vi "D-O Module (Main).vi"(7 "Name of Parent Panel":string="Main.vi", 9 "New Center Coords":T1={"Horizontal"=470, "Vertical"=200}, 10 "Config":variant, 11 "Main UI Message Queue":refnum<queue>) -> ()   [LabVIEW 2018, in "D-O Module.lvlib"]
doc: "This Continuous Measurement sample project is based on the Queued Message Handler template.\n\nThe Event Handling Loop generates messages based on user interface actions.\n\nThe Message Handling Loop processes messages generated by the Event Handling Loop, or by other messages. There are also Acquisition and Logging message handling loop subVIs, and a chart updating loop."
uses:
  D-O Module.lvlib
  support/Message Queue/Message Cluster.ctl
  <vilib>/Utility/miscctls.llb/LVPoint32TypeDef.ctl
  controls/UI Data.ctl
  controls/UI State.ctl
  D-O Module State Cluster.ctl
  D-O Module Config Cluster.ctl
  Valve Clusters.ctl
  D-O Module Settings Cluster.ctl
  D-O Device Settings Cluster.ctl
  VICI Electronic Actuator/VICI Electronic Actuator Settings.ctl
  Measure Instrument/State Enum.ctl
  D-O Module Display.ctl
  Sequencing/Squence Update Cluster.ctl
  support/Message Queue/Enqueue Message (Single).vi
  <vilib>/Utility/error.llb/Error Cluster From Error Code.vi
  <vilib>/ErrorRing/Error Ring.xnode
  support/User Event - Stop/User Event - Stop.lvlib
  support/Support Library.lvlib
  support/Message Queue/Message Queue.lvlib
  Measure Instrument/D-O Module Engine.lvlib
  Measure Instrument/Feed Module Engine.lvlib
  Sequencing/Sequencing Library.lvlib
  D-O Settings Dialog.vi
  support/Command Log VIs/Command Logging.lvlib
  DIO Valve/VICI Electronic Actuator.lvlib
panel:
  out "Sequence Started":bool
  in  "Settings Button":bool
  out "ScanCode":i16
  out "Ring":u16(ring)=2
  out "Log File path":path
  out "Status":string
  in  "Exit":bool
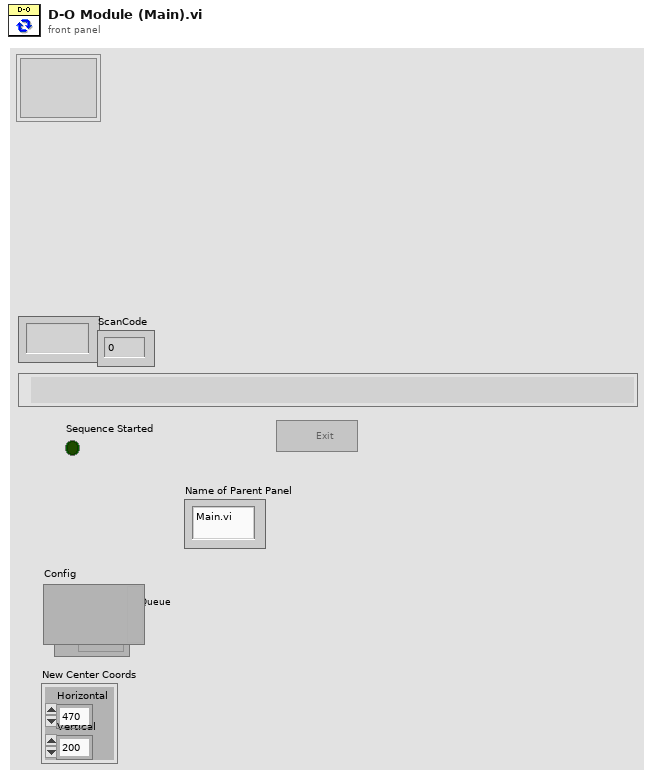
[diagram p1: front panel]
types:
  T1 = typedef "LVPoint32TypeDef.ctl" = cluster{"Horizontal":i32, "Vertical":i32}
  T2 = typedef "D-O Module.lvlib/D-O Module Config Cluster.ctl" = cluster{"GUID":string, "Drop Coords":T1, "Process Name":string, "Queue Name":string, "Settings":T3, "Load Count":i32}
  T3 = typedef "D-O Module.lvlib/Valve Clusters.ctl" = cluster{"Valve Settings":T4, "Valve Type":enum16{"Default", "Digital Output Valve", "VICI Electronic Actuator"}, "Time On (Sec)":dbl, "Time Off (Sec)":dbl, "Run?":bool}
  T4 = typedef "D-O Module.lvlib/D-O Module Settings Cluster.ctl" = cluster{"D-O Settings":T5, "VICI Electronic Actuator":T6}
  T5 = typedef "D-O Module.lvlib/D-O Device Settings Cluster.ctl" = cluster{"DAQmx Task Name":refnum<k21>, "Output Channel":u16, "Output Channel Names":string[]}
  T6 = typedef "VICI Electronic Actuator.lvlib/VICI Electronic Actuator Settings.ctl" = cluster{"VISA resource name":refnum<visa-resource-name>, "Mode":enum16{"Two Positions With Stops", "Two Positions Without Stops", "Mutiposition"}, "Simulated":bool}
  T7 = typedef "D-O Module.lvlib/D-O Module State Cluster.ctl" = cluster{"D-O Module Config":T2, "State":T8, "Start Time":timestamp, "Current Time":timestamp, "First Iteration":bool, "Data":cluster{"Valve State":T4}, "Process Name":string, "Queue Name":string, "Program On?":bool}
  T8 = typedef "Feed Module.lvlib/Feed Module Engine.lvlib/State Enum.ctl" = enum16{"Measuring", "Idle", "Paused"}
  T9 = typedef "UI State.ctl" = enum16{"Idle", "Acquiring and Logging", "Waiting for Exit", "Waiting for Exit (Acq Stopped)", "Waiting for Exit (Log Stopped)", "Waiting for Stop", "Waiting for Stop (Acq Stopped)", "Waiting for Stop (Log Stopped)"}
  T10 = typedef "UI Data.ctl" = cluster{"Start Ref":refnum<vi>, "Trigger Ref":refnum<vi>, "Stop Ref":refnum<vi>, "Settings Ref":refnum<vi>, "Status Ref":refnum<vi>, "Exit Ref":refnum<vi>, "Data Ref":refnum<vi>}
  T11 = typedef "D-O Module.lvlib/All Message Queues.ctl" = cluster{"Engine":refnum<queue>, "D-O UI":refnum<queue>, "D-O Engine":refnum<queue>, "D-O Display":refnum<queue>}
  T12 = typedef "Sequencing Library.lvlib/Squence Update Cluster.ctl" = cluster{"Auto?":bool, "Manual Entry":dbl, "Setpoint":dbl}
  T13 = enum8{"Enabled", "Disabled", "Disabled and Grayed Out"}
  T14 = typedef "D-O Module.lvlib/D-O Module Display.ctl" = cluster{"D-O State ":u16, "Cycle Period":dbl}
  T15 = cluster{"Shift":bool, "Ctrl":bool, "Alt":bool, "Cmd":bool, "Opt":bool}
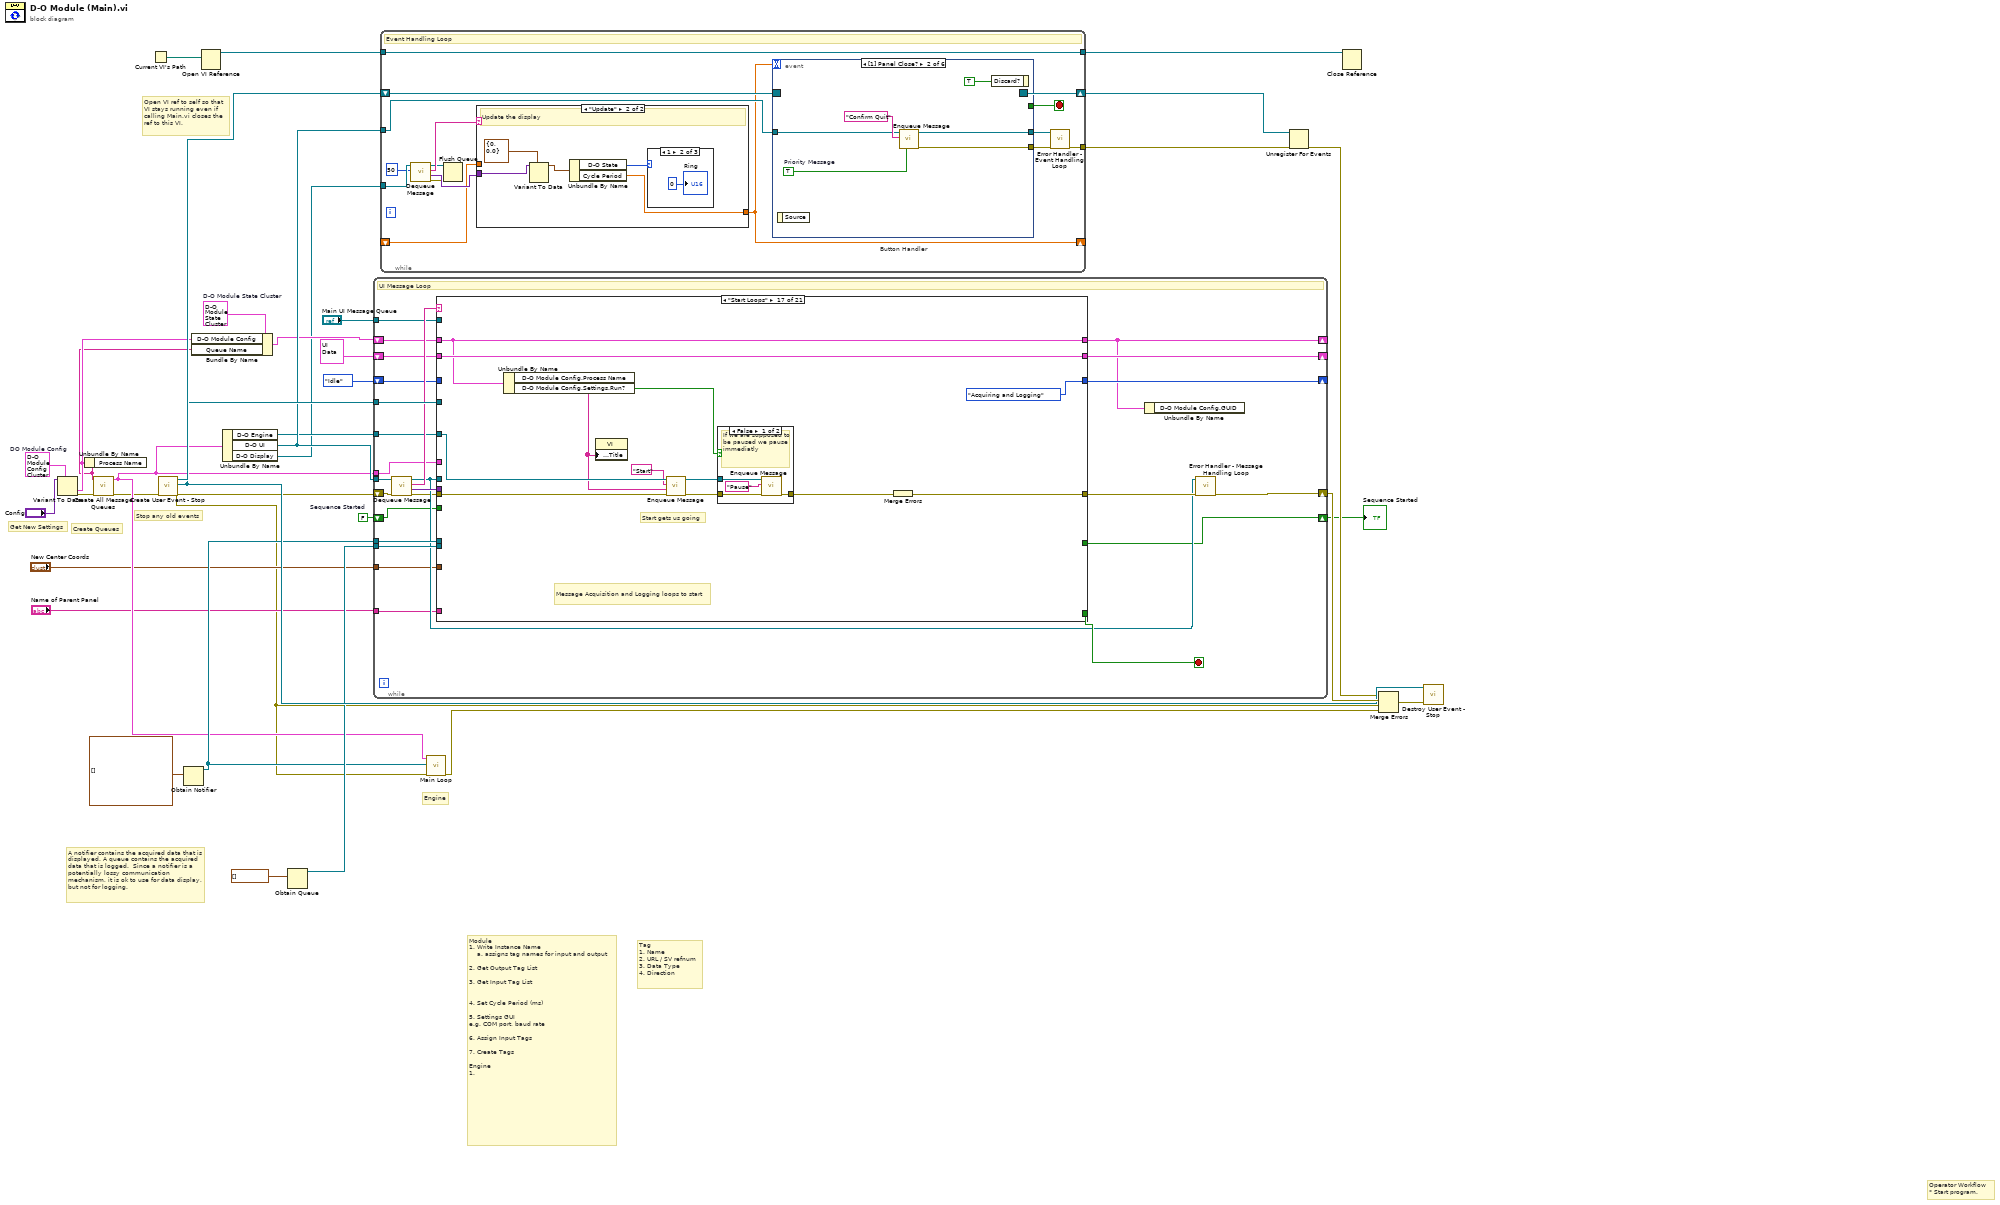
[diagram p0: block diagram]
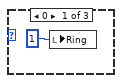
[diagram p3: hidden frame]
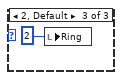
[diagram p4: hidden frame]
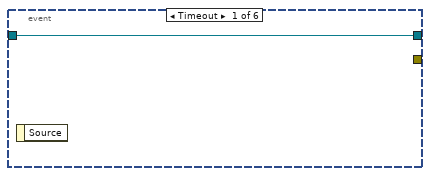
[diagram p5: hidden frame]
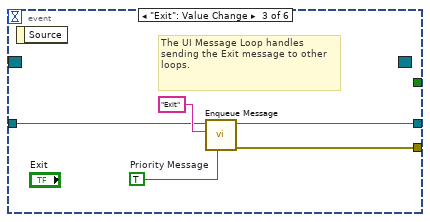
[diagram p6: hidden frame]
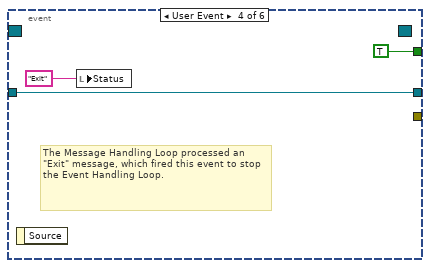
[diagram p7: hidden frame]
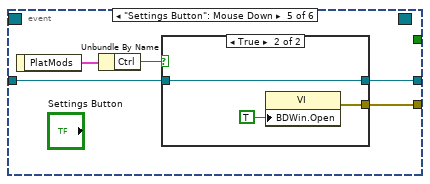
[diagram p8: hidden frame]
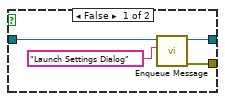
[diagram p9: hidden frame]
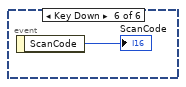
[diagram p10: hidden frame]
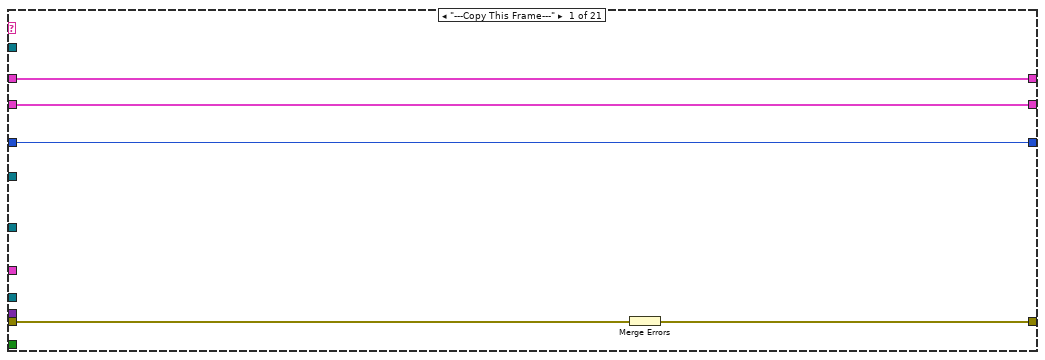
[diagram p11: hidden frame]
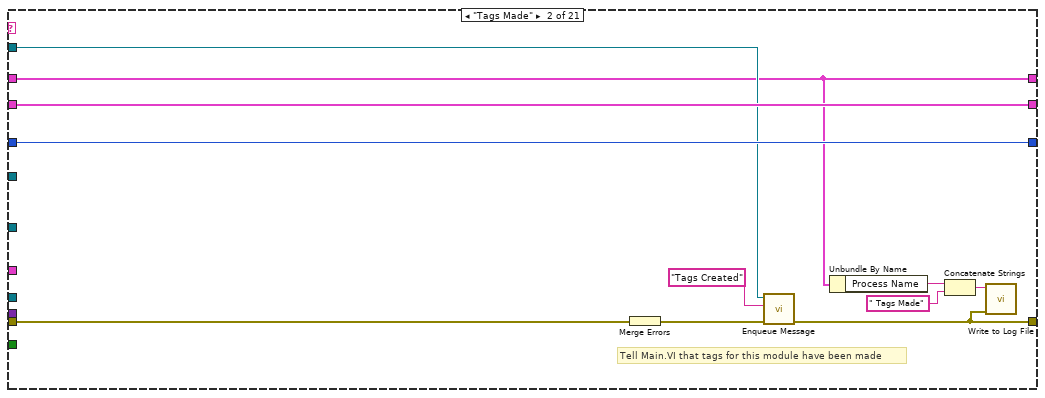
[diagram p12: hidden frame]
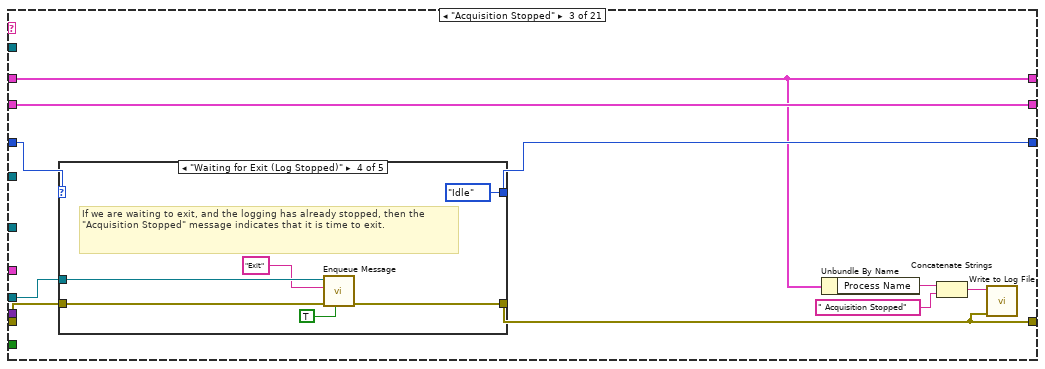
[diagram p13: hidden frame]
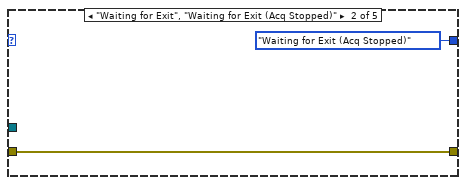
[diagram p15: hidden frame]
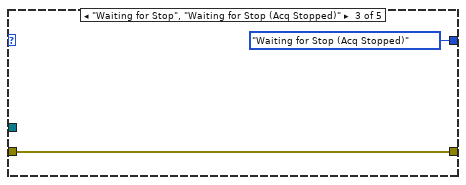
[diagram p16: hidden frame]
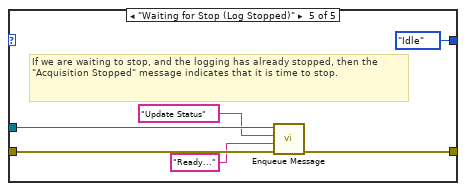
[diagram p17: hidden frame]
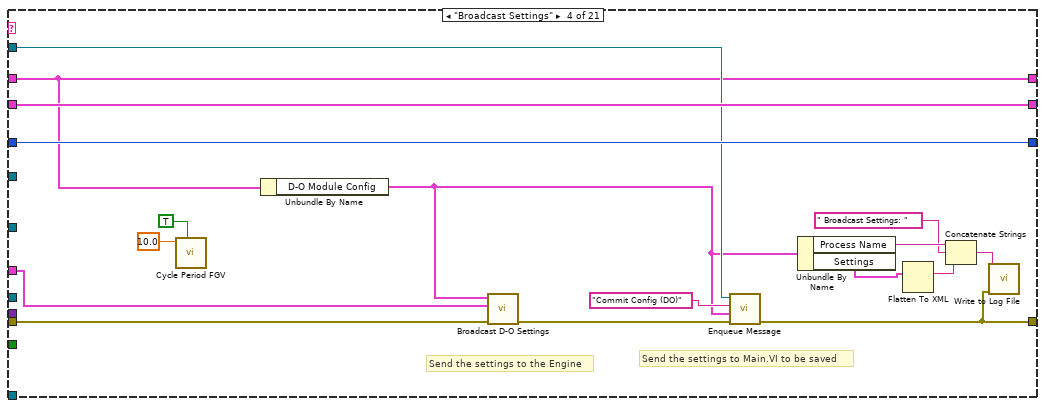
[diagram p18: hidden frame]
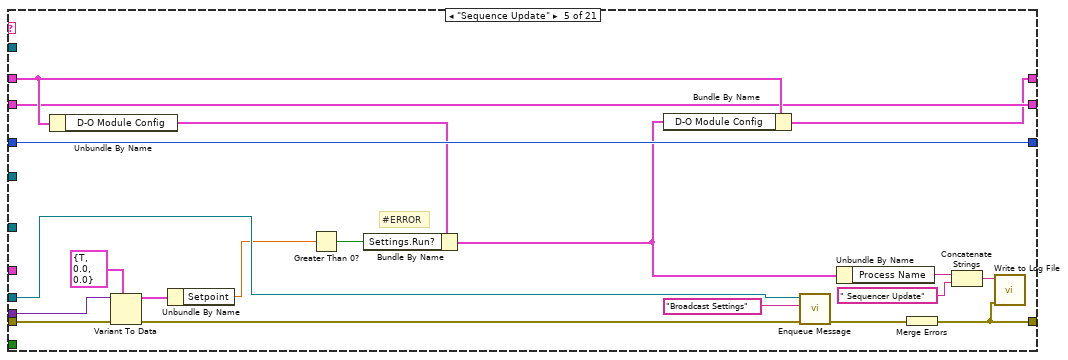
[diagram p19: hidden frame]
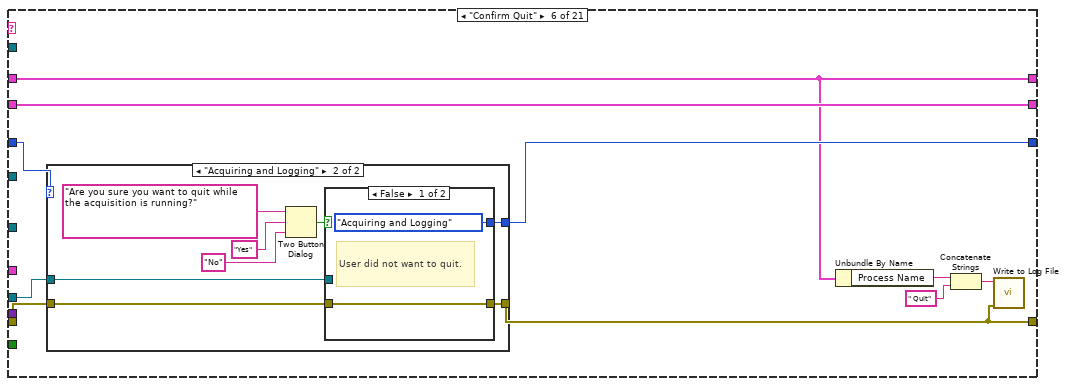
[diagram p20: hidden frame]
diagram:
  w7 = FALSE  # Sequence Started
  w6 = T2 {"GUID"="", "Drop Coords"={"Horizontal"=0, "Vertical"=0}, "Process Name"="", "Queue Name"="", "Settings"={"Valve Settings"={"D-O Settings"={"DAQmx Task Name"="", "Output Channel"=0, "Output Channel Names"=[]}, "VICI Electronic Actuator"={"VISA resource name"="", "Mode"=enum."Two Positions With Stops", "Simulated"=FALSE}}, "Valve Type"=enum."Default", "Time On (Sec)"=0.0, "Time Off (Sec)"=0.0, "Run?"=FALSE}, "Load Count"=0}  # DO Module Config
  w14 = T7 {"D-O Module Config"={"GUID"="", "Drop Coords"={"Horizontal"=0, "Vertical"=0}, "Process Name"="", "Queue Name"="", "Settings"={"Valve Settings"={"D-O Settings"={"DAQmx Task Name"="", "Output Channel"=0, "Output Channel Names"=[]}, "VICI Electronic Actuator"={"VISA resource name"="", "Mode"=enum."Two Positions With Stops", "Simulated"=FALSE}}, "Valve Type"=enum."Digital Output Valve", "Time On (Sec)"=0.0, "Time Off (Sec)"=0.0, "Run?"=FALSE}, "Load Count"=0}, "State"=enum."Idle", "Start Time"=timestamp(0 s since 1904-01-01), "Current Time"=timestamp(0 s since 1904-01-01), "First Iteration"=FALSE, "Data"={"Valve State"={"D-O Settings"={"DAQmx Task Name"="", "Output Channel"=0, "Output Channel Names"=[]}, "VICI Electronic Actuator"={"VISA resource name"="", "Mode"=enum."Two Positions With Stops", "Simulated"=FALSE}}}, "Process Name"="", "Queue Name"="", "Program On?"=FALSE}  # D-O Module State Cluster
  # "Stop any old events"
  # "Create Queues"
  # "Get New Settings"
  # "Open VI ref to self so that\nVI stays running even if\ncalling Main.vi closes the\nref to this VI."
  # "Engine"
  # "Operator Workflow\n* Start program."
  # "Module \n1. Write Instance Name\n    a. assigns tag names for input and output\n\n2. Get Output Tag List\n\n3. Get Input Tag List\n\n\n4. Set Cycle Period (ms)\n\n5. Settings GUI\ne.g. COM port, baud rate\n\n6. Assign Input Tags\n\n7. Create Tags\n\nEngine\n1."
  # "Tag\n1. Name\n2. URL / SV refnum\n3. Data Type\n4. Direction"
  # "A notifier contains the acquired data that is displayed. A queue contains the acquired data that is logged.  Since a notifier is a potentially lossy communication mechanism, it is ok to use for data display, but not for logging."
  n1 = Variant To Data(type=w6, Variant="Config") -> (data=w5:T2, error out=w4:errorcluster)  [unwired: 1 in]
  n2 = Unbundle By Name(w5) -> ("Process Name"=w1:string)
  n3 = call "Create All Message Queues.vi"("error in (no error)"=w4, "Process Name"=w1) -> ("error out"=w3:errorcluster, "Message Queues"=w11:T11)  [unwired: 8 in]
  n4 = Current VI's Path() -> (path=w17:path)
  n5 = call "Create User Event - Stop.vi"("error in (no error)"=w3) -> ("error out"=w2:errorcluster, "User Event - Stop"=w31:refnum<user-event>, "Stop Event Registration Refnum"=w32:refnum<event-registration>)  [unwired: 8 in]
  n6 = Obtain Notifier(notification data type=waveform(dbl)[] []) -> (notifier out=w20:refnum<notifier>)  [unwired: 3 in, 2 out]
  n7 = Bundle By Name(cluster=w14, "D-O Module Config"=w5, "Queue Name"=w1) -> (w16:T7)
  n8 = Open VI Reference(vi path=w17) -> (vi reference=w18:refnum<vi>)  [unwired: 5 in, 1 out]
  n9 = Unbundle By Name(w11) -> ("D-O Engine"=w23:refnum<queue>, "D-O UI"=w27:refnum<queue>, "D-O Display"=w13:refnum<queue>)
  n10 = Obtain Queue(element data type=waveform(dbl)[] []) -> (queue out=w22:refnum<queue>)  [unwired: 4 in, 2 out]
  n11 = while {
    tunnel: w27 -> [w55]
    tunnel: w31 -> [w59]
    shift-right: [w49] -> w35
    shift-left: w2 -> [w58]
    shift-right: [w36] -> _
    shift-left: w16 -> [w43]
    shift-right: [w53] -> _
    shift-left: T10 {"Start Ref"=refnum, "Trigger Ref"=refnum, "Stop Ref"=refnum, "Settings Ref"=refnum, "Status Ref"=refnum, "Exit Ref"=refnum, "Data Ref"=refnum} ("Measurement UI Controls") -> [w54]
    tunnel: w20 -> [w52]
    tunnel: w22 -> [w51]
    shift-right: [w46] -> _
    shift-left: UI_State."Idle" ("UI State") -> [w47]
    tunnel: w23 -> [w45]
    tunnel: "Main UI Message Queue" -> [w42]
    tunnel: w11 -> [w41]
    tunnel: "New Center Coords" -> [w40]
    tunnel: "Name of Parent Panel" -> [w39]
    shift-right: [w38] -> w8
    shift-left: w7 -> [w37]
    stop <- w60 stop-if-true
    # "UI Message Loop"
    n12 = call "Dequeue Message.vi"("error in (no error)"=w58, "Message Queue"=w55) -> ("error out"=w44:errorcluster, "Message Data"=w56:variant, "Message"=w57:string, "dup Message Queue"=w48:refnum<queue>)  [unwired: 6 in]
    n13 = case "Message Cases" shown="\"Start Loops\"" w57 {
      selector: w57 -> [_ _ _ _ _ _ _ _ _ _ _ _ _ _ _ _ _ _ _ _ w480]
      tunnel: w48 -> [_ _ w82 _ w137 w149 _ w207 w222 w249 _ w283 w302 w308 w344 w376 _ _ w436 _ _]
      tunnel: w44 -> [w65 w76 w83 w118 w135 w148 w175 w188 w226 w253 w268 w278 w299 w310 w342 w375 w402 w418 w438 w471 _]
      tunnel: [w64 w70 w81 w111 w123 w143 w176 w182 w216 w228 w268 w273 w294 w309 w333 w364 w406 w416 w433 w472 w483] -> w50
      tunnel: [_ _ _ _ _ _ _ _ _ TRUE _ _ _ _ _ _ _ _ _ _ _] -> w60
      tunnel: w56 -> [_ _ _ _ w138 _ w178 _ w225 w237 _ _ _ _ _ _ _ _ _ w470 _]
      tunnel: w59 -> [_ _ _ _ _ _ _ _ _ w252 _ _ _ _ _ _ _ _ _ _ _]
      tunnel: w43 -> [w61 w66 w77 w115 w140 w142 w173 w186 w213 w229 w259 w269 w301 w307 w338 w371 w400 w412 w440 w461 w478]
      tunnel: w54 -> [w63 w75 w86 w121 w139 w151 w180 w204 w227 w250 w267 w279 w306 w313 w339 w372 w405 w423 w456 w467 w485]
      tunnel: [w63 w75 w86 w121 w139 w151 w180 w204 w227 w250 w266 w279 w306 w313 w339 w372 w405 w423 w456 w467 w485] -> w53
      tunnel: w52 -> [_ _ _ _ _ _ _ _ _ w248 _ _ _ _ _ _ _ _ _ _ _]
      tunnel: w51 -> [_ _ _ _ _ _ _ _ _ w244 _ _ _ _ _ _ _ _ _ _ _]
      tunnel: w47 -> [w62 w74 w85 w120 w141 w150 w174 w193 w217 _ _ _ w305 w312 _ _ _ _ w445 w462 w484]
      tunnel: [w62 w74 w84 w120 w141 w147 w174 w194 w217 UI_State."Idle" ("UI State") UI_State."Idle" ("UI State") UI_State."Idle" ("UI State") w305 w311 UI_State."Acquiring and Logging" ("UI State") UI_State."Acquiring and Logging" ("UI State") UI_State."Acquiring and Logging" ("UI State") UI_State."Acquiring and Logging" ("UI State") w446 w462 w484] -> w46
      tunnel: w45 -> [_ _ _ _ _ _ _ w192 _ w236 _ _ _ _ _ _ w403 w421 w444 _ _]
      tunnel: w42 -> [_ w71 _ w117 _ _ _ _ _ w238 _ _ _ _ _ _ _ _ _ _ _]
      tunnel: [w61 w66 w77 w115 w136 w142 w173 w181 w213 w229 w259 w269 w290 w307 w332 w361 w400 w412 w429 w461 w478] -> w36
      tunnel: w41 -> [_ _ _ w113 _ _ _ _ _ _ _ _ w296 _ _ _ _ _ _ _ _]
      tunnel: w40 -> [_ _ _ _ _ _ _ _ _ _ _ w276 _ _ _ _ _ _ _ _ _]
      tunnel: w39 -> [_ _ _ _ _ _ _ _ _ _ _ w275 _ _ _ _ _ _ _ _ _]
      tunnel: [_ _ _ _ _ _ _ _ _ _ _ _ _ _ _ w369 _ _ _ _ _] -> w38
      tunnel: w37 -> [_ _ _ _ _ _ _ _ _ _ _ _ _ _ _ w365 _ _ _ _ _]
      frame "---Copy This Frame---" {
        # "Duplicate this frame when creating new messages.  Change this comment in the duplicated frame to describe this message."
        n14 = Merge Errors(w65) -> (w64:errorcluster)
      }
      frame "Tags Made" {
        # "Tell Main.VI that tags for this module have been made"
        # "Duplicate this frame when creating new messages.  Change this comment in the duplicated frame to describe this message."
        n15 = Merge Errors(w76) -> (w72:errorcluster)
        n16 = call-poly "Enqueue Message.vi"("error in (no error)"=w72, "Message"="Tags Created", "Message Queue"=w71) -> ("error out"=w70:errorcluster)  [unwired: 7 in, 1 out]
        n17 = Unbundle By Name(w66) -> ("Process Name"=w69:string)
        n18 = Concatenate Strings(w69, " Tags Made" ("text")) -> (w67:string)
        n19 = call "Write to Log File.vi"("error in"=w70, "text"=w67) -> ()  [unwired: 9 in, 1 out]
      }
      frame "Acquisition Stopped" {
        # "Logic for determining what action to take when the acquisition has stopped."
        n20 = case shown="\"Waiting for Exit (Log Stopped)\"" w85 {
          selector: w85 -> [w88 _ _ _ _]
          tunnel: [w88 UI_State."Waiting for Exit (Acq Stopped)" ("UI State") UI_State."Waiting for Stop (Acq Stopped)" ("UI State") UI_State."Idle" ("UI State") UI_State."Idle" ("UI State")] -> w84
          tunnel: w83 -> [w87 w89 w91 w97 w103]
          tunnel: [w87 w89 w91 w96 w102] -> w81
          tunnel: w82 -> [_ _ _ w95 w101]
          frame Default {
          }
          frame "Waiting for Exit", "Waiting for Exit (Acq Stopped)" {
          }
          frame "Waiting for Stop", "Waiting for Stop (Acq Stopped)" {
          }
          frame "Waiting for Exit (Log Stopped)" {
            # "If we are waiting to exit, and the logging has already stopped, then the \"Acquisition Stopped\" message indicates that it is time to exit."
            n21 = call-poly "Enqueue Message.vi"("Priority Message? (F)"=TRUE, "error in (no error)"=w97, "Message"="Exit", "Message Queue"=w95) -> ("error out"=w96:errorcluster)  [unwired: 6 in, 1 out]
          }
          frame "Waiting for Stop (Log Stopped)" {
            # "If we are waiting to stop, and the logging has already stopped, then the \"Acquisition Stopped\" message indicates that it is time to stop."
            n22 = call-poly "Enqueue Message.vi"("error in (no error)"=w103, "Message Data"="Ready..." ("Message"), "Message"="Update Status", "Message Queue"=w101) -> ("error out"=w102:errorcluster)  [unwired: 6 in, 1 out]
          }
        }
        n23 = Unbundle By Name(w77) -> ("Process Name"=w80:string)
        n24 = Concatenate Strings(w80, " Acquisition Stopped" ("text")) -> (w78:string)
        n25 = call "Write to Log File.vi"("error in"=w81, "text"=w78) -> ()  [unwired: 9 in, 1 out]
      }
      frame "Broadcast Settings" {
        # "Send the settings to Main.VI to be saved"
        # "Send the settings to the Engine"
        # "Send the 'Update Settings' message to the Logging and Acquisition message loops."
        n26 = call "Cycle Period FGV.vi"("Write"=TRUE, "Cycle Period In (ms)"=10.0) -> ()  [unwired: 8 in, 2 out]
        n27 = Unbundle By Name(w115) -> ("D-O Module Config"=w107:T2)
        n28 = call "Broadcast D-O Settings.vi"("error in (no error)"=w118, "Message Queues"=w113, "D-O Module Config"=w107) -> ("error out"=w116:errorcluster)  [unwired: 8 in]
        n29 = call-poly "Enqueue Message.vi"("error in (no error)"=w116, "Message Data"=w107, "Message"="Commit Config (DO)", "Message Queue"=w117) -> ("error out"=w111:errorcluster)  [unwired: 6 in, 1 out]
        n30 = Unbundle By Name(w107) -> ("Process Name"=w110:string, "Settings"=w105:T3)
        n31 = Flatten To XML(anything=w105) -> (xml string=w106:string)
        n32 = Concatenate Strings(w110, " Broadcast Settings: " ("text"), w106) -> (w108:string)
        n33 = call "Write to Log File.vi"("error in"=w111, "text"=w108) -> ()  [unwired: 9 in, 1 out]
      }
      frame "Sequence Update" {
        # "#ERROR"
        n34 = Unbundle By Name(w140) -> ("D-O Module Config"=w134:T2)
        n35 = Variant To Data(error in=w135, type=T12 {"Auto?"=TRUE, "Manual Entry"=0.0, "Setpoint"=0.0} ("Cluster"), Variant=w138) -> (data=w132:T12, error out=w129:errorcluster)
        n36 = Unbundle By Name(w132) -> ("Setpoint"=w127:dbl)
        n37 = Greater Than 0?(x=w127) -> (x > 0?=w128:bool)
        n38 = Bundle By Name(cluster=w134, "Settings.Run?"=w128) -> (w122:T2)
        n39 = Bundle By Name(cluster=w140, "D-O Module Config"=w122) -> (w136:T7)
        n40 = call-poly "Enqueue Message.vi"("error in (no error)"=w129, "Message"="Broadcast Settings", "Message Queue"=w137) -> ("error out"=w131:errorcluster)  [unwired: 7 in, 1 out]
        n41 = Unbundle By Name(w122) -> ("Process Name"=w126:string)
        n42 = Merge Errors(w131) -> (w123:errorcluster)
        n43 = Concatenate Strings(w126, " Sequencer Update" ("text")) -> (w124:string)
        n44 = call "Write to Log File.vi"("error in"=w123, "text"=w124) -> ()  [unwired: 9 in, 1 out]
      }
      frame "Confirm Quit" {
        # "Confirm Quit - Message that can confirm whether or not the user wants to exit the application."
        n45 = case shown="\"Acquiring and Logging\"" w150 {
          tunnel: w149 -> [w156 w162]
          tunnel: w148 -> [w155 w160]
          tunnel: [w152 w159] -> w143
          tunnel: [UI_State."Idle" ("UI State") w158] -> w147
          frame Default {
            # "If 'Confirm Quit' comes in while the system is idle, there is no need for a confirmation message."
            n46 = call-poly "Enqueue Message.vi"("Priority Message? (F)"=TRUE, "error in (no error)"=w155, "Message"="Exit", "Message Queue"=w156) -> ("error out"=w152:errorcluster)  [unwired: 6 in, 1 out]
          }
          frame "Acquiring and Logging" {
            n47 = Two Button Dialog(message="Are you sure you want to quit while the acquisition is running?" ("Confirm Quit Message"), 1:"No" ("No"), 2:"Yes" ("Yes")) -> (T button?=w161:bool)
            n48 = case shown="False" w161 {
              tunnel: w162 -> [_ w172]
              tunnel: w160 -> [w166 w171]
              tunnel: [w166 w170] -> w159
              tunnel: [UI_State."Acquiring and Logging" ("UI State") UI_State."Waiting for Exit" ("UI State")] -> w158
              frame False {
                # "User did not want to quit."
              }
              frame True {
                n49 = call-poly "Enqueue Message.vi"("error in (no error)"=w171, "Message"="Stop", "Message Queue"=w172) -> ("error out"=w170:errorcluster)  [unwired: 7 in, 1 out]
              }
            }
          }
        }
        n50 = Unbundle By Name(w142) -> ("Process Name"=w146:string)
        n51 = Concatenate Strings(w146, " Quit" ("text")) -> (w144:string)
        n52 = call "Write to Log File.vi"("error in"=w143, "text"=w144) -> ()  [unwired: 9 in, 1 out]
      }
      frame "Display Log File Path" {
        n53 = Variant To Data(error in=w175, type=path "", Variant=w178) -> (data=→"Log File path":path, error out=w176:errorcluster)
      }
      frame "E-Stop" {
        # "Pause the DO when E-Stop is sent"
        # "Message Acquisition and Logging loops to stop"
        # "Enable: Start, Exit, Settings\nDisable: Stop"
        # "Stop the pumps."
        n54 = Unbundle By Name(w204) -> ("Trigger Ref"=w195:refnum<vi>, "Stop Ref"=w196:refnum<vi>, "Start Ref"=w199:refnum<vi>, "Exit Ref"=w198:refnum<vi>, "Settings Ref"=w197:refnum<vi>)
        n55 = call-poly "Enqueue Message.vi"("error in (no error)"=w188, "Message Data"="Ready..." ("Ready..."), "Message"="Update Status", "Message Queue"=w207) -> ("error out"=w190:errorcluster)  [unwired: 6 in, 1 out]
        n56 = Build Array(w199, w198, w197) -> (w202:refnum<vi>[])
        n57 = Build Array(w195, w196) -> (w201:refnum<vi>[])
        n58 = call-poly "Enqueue Message.vi"("error in (no error)"=w190, "Message"="Pause", "Message Queue"=w192) -> ("error out"=w189:errorcluster)  [unwired: 7 in, 1 out]
        n59 = call "Set Enable State on Multiple Controls.vi"("Enable?"=FALSE, "Controls"=w201) -> ()  [unwired: 10 in]
        n60 = call "Set Enable State on Multiple Controls.vi"("Enable?"=TRUE, "Controls"=w202) -> ()  [unwired: 10 in]
        n61 = case shown="Default" w193 {
          selector: w193 -> [_ w209]
          tunnel: [UI_State."Waiting for Stop" ("UI State") w209] -> w194
          frame Default {
          }
          frame "Waiting for Exit" {
          }
        }
        n62 = Merge Errors(w189) -> (w182:errorcluster)
        n63 = Bundle By Name(cluster=w186, "State"=State_Enum."Idle") -> (w181:T7)
        n64 = Unbundle By Name(w181) -> ("Process Name"=w185:string)
        n65 = Concatenate Strings(w185, " E-STOP" ("text")) -> (w183:string)
        n66 = call "Write to Log File.vi"("error in"=w182, "text"=w183) -> ()  [unwired: 9 in, 1 out]
      }
      frame "Error" {
        # "Error - Check the error message data and respond accordingly. This message is sent by the \"Error Handler\" VIs at the end of each loop in this application."
        n67 = Variant To Data(error in=w226, type=errorcluster {"status"=FALSE, "code"=0, "source"=""} ("error out"), Variant=w225) -> (data=w223:errorcluster, error out=w219:errorcluster)
        n68 = call <vilib>:"Simple Error Handler.vi"("error in (no error)"=w223) -> ()  [unwired: 4 in, 5 out]
        n69 = call-poly "Enqueue Message.vi"("Priority Message? (F)"=TRUE, "Message"="Exit", "Message Queue"=w222) -> ("error out"=w218:errorcluster)  [unwired: 7 in, 1 out]
        n70 = Merge Errors(w218, w219) -> (w216:errorcluster)
        n71 = Unbundle By Name(w213) -> ("Process Name"=w215:string)
        n72 = call <vilib>:"General Error Handler.vi"("error in (no error)"=w216) -> ("message"=w211:string, "error out"=w210:errorcluster)  [unwired: 10 in, 3 out]
        n73 = Concatenate Strings(w215, " Error: " ("text"), w211) -> (w214:string)
        n74 = call "Write to Log File.vi"("error in"=w210, "text"=w214) -> ()  [unwired: 9 in, 1 out]
      }
      frame "Exit" {
        w241 = TRUE  # Delete Module?
        # "Stop DO Engine then Close it"
        # "Don't check the error outs. The acquisition and logging queues may have already been released."
        # "Close references owned by the Main VI."
        # "Stop the VI"
        # "Exit - Fire the User Event to stop the Event Handling Loop.  Also send Exit messages to the Acquisition and Logging loops."
        n75 = Release Queue(queue=w249, error in (no error)=w253) -> (error out=w247:errorcluster)  [unwired: 1 in, 2 out]
        n76 = call "Fire User Event - Stop.vi"("User Event - Stop"=w252) -> ("error out"=w251:errorcluster)  [unwired: 10 in]
        n77 = Release Notifier(notifier=w248, error in (no error)=w247) -> (error out=w246:errorcluster)  [unwired: 1 in, 2 out]
        n78 = Release Queue(queue=w244, error in (no error)=w246) -> (error out=w245:errorcluster)  [unwired: 1 in, 2 out]
        n79 = call-poly "Enqueue Message.vi"("Message"="Stop", "Message Queue"=w236) -> ("dup Message Queue"=w234:refnum<queue>)  [unwired: 8 in, 1 out]
        n80 = Variant To Data(type=w241, Variant=w237) -> (data=w240:bool, error out=w242:errorcluster)  [unwired: 1 in]
        n81 = Select(t=w241, s=w242, f=w240) -> (s? t:f=w239:bool)
        n82 = call-poly "Enqueue Message.vi"("Message"="Exit", "Message Queue"=w234) -> ()  [unwired: 8 in, 2 out]
        n83 = case "Don't enqueue Delete Module if opening campaign because it\nwill already have been deleted and new config loaded and we create\na race condition." shown="True" w239 {
          tunnel: w238 -> [_ w257]
          tunnel: w229 -> [_ w256]
          frame False {
          }
          frame True {
            n84 = Unbundle By Name(w256) -> ("D-O Module Config.GUID"=w255:string)
            n85 = call-poly "Enqueue Message.vi"("Message Data"=w255, "Message"="Delete Module", "Message Queue"=w257) -> ()  [unwired: 7 in, 2 out]
          }
        }
        n86 = Merge Errors(w251, w245) -> (w228:errorcluster)
        n87 = Unbundle By Name(w229) -> ("Process Name"=w232:string)
        n88 = Concatenate Strings(w232, " Exit" ("text")) -> (w230:string)
        n89 = call "Write to Log File.vi"("error in"=w228, "text"=w230) -> ()  [unwired: 9 in, 1 out]
      }
      frame "Init UI Refs" {
        # "Enable: Start, Exit, Settings\nDisable: Stop"
        # "Init UI Refs - Store control references for UI controls.  Also enable/disable controls appropriately."
        n90 = property class="VI"("Front Panel.Closeable"=TRUE ("Front Panel Window:Closeable")) -> ()  [unwired: 2 in, 2 out]
        n91 = control-ref of="Status"() -> (w264:refnum<vi>)
        n92 = control-ref of="Exit"() -> (w261:refnum<vi>)
        n93 = Bundle By Name(cluster=w267, "Status Ref"=w264, "Exit Ref"=w261) -> (w266:T10)
        n94 = Build Array(w261) -> (w263:refnum<vi>[])
        n95 = call "Set Enable State on Multiple Controls.vi"("Enable?"=TRUE, "Controls"=w263) -> ()  [unwired: 10 in]
      }
      frame "Initialize" {
        # "Initialize - Get configuration settings, then message the UI to initialize, and broadcast the settings to the other message loops."
        n96 = Unbundle By Name(w269) -> ("Process Name"=w274:string)
        n97 = property class="VI" props=["FP.State"]() -> (reference out=w277:refnum<vi>)  [unwired: 2 in, 2 out]
        n98 = call-poly "Enqueue Message.vi"("error in (no error)"=w278, "Message"="Init UI Refs", "Message Queue"=w283) -> ("error out"=w281:errorcluster, "dup Message Queue"=w282:refnum<queue>)  [unwired: 7 in]
        n99 = call "Make Child and Move.vi"("Process Name"=w274, "Name of Parent Panel"=w275, "New Center Coords"=w276, "VI in"=w277) -> ()  [unwired: 8 in]
        n100 = call-poly "Enqueue Message.vi"("error in (no error)"=w281, "Message"="Broadcast Settings", "Message Queue"=w282) -> ("error out"=w289:errorcluster, "dup Message Queue"=w288:refnum<queue>)  [unwired: 7 in]
        n101 = call-poly "Enqueue Message.vi"("error in (no error)"=w289, "Message Data"="Ready..." ("Ready..."), "Message"="Update Status", "Message Queue"=w288) -> ("error out"=w273:errorcluster)  [unwired: 6 in, 1 out]
        n102 = Unbundle By Name(w269) -> ("Process Name"=w272:string)
        n103 = Concatenate Strings(w272, " Initialize" ("text")) -> (w270:string)
        n104 = call "Write to Log File.vi"("error in"=w273, "text"=w270) -> ()  [unwired: 9 in, 1 out]
      }
      frame "Launch Settings Dialog" {
        # "Keep track of whether the Dialog has been opened."
        # "Launch the Settings Dialog when the user clicks the 'Settings' button."
        n105 = Unbundle By Name(w301) -> ("D-O Module Config.Load Count"=w303:i32)
        n106 = Increment(x=w303) -> (x+1=w304:i32)
        n107 = Bundle By Name(cluster=w301, "D-O Module Config.Load Count"=w304) -> (w297:T7)
        n108 = call-by-ref "?"("error in (no error)"=w299, "Message Queues"=w296, "D-O Module State Cluster In"=w297) -> ("error out"=w295:errorcluster, "D-O Module Config Out"=w298:T2)  [unwired: 7 in, 4 out]
        n109 = Bundle By Name(cluster=w301, "D-O Module Config"=w298) -> (w290:T7)
        n110 = call-poly "Enqueue Message.vi"("error in (no error)"=w295, "Message"="Broadcast Settings", "Message Queue"=w302) -> ("error out"=w294:errorcluster)  [unwired: 7 in, 1 out]
        n111 = Unbundle By Name(w290) -> ("Process Name"=w293:string)
        n112 = Concatenate Strings(w293, "Launch Settings Dialog" ("text")) -> (w291:string)
        n113 = call "Write to Log File.vi"("error in"=w294, "text"=w291) -> ()  [unwired: 9 in, 1 out]
      }
      frame "Logging Stopped" {
        # "Logic for determining what action to take when the logging has stopped."
        n114 = case shown="\"Waiting for Exit (Acq Stopped)\"" w312 {
          selector: w312 -> [w315 _ _ _ _]
          tunnel: [w315 UI_State."Waiting for Exit (Log Stopped)" ("UI State") UI_State."Waiting for Stop (Log Stopped)" ("UI State") UI_State."Idle" ("UI State") UI_State."Idle" ("UI State")] -> w311
          tunnel: w310 -> [w314 w316 w318 w324 w330]
          tunnel: [w314 w316 w318 w323 w329] -> w309
          tunnel: w308 -> [_ _ _ w322 w328]
          frame Default {
          }
          frame "Waiting for Exit", "Waiting for Exit (Log Stopped)" {
          }
          frame "Waiting for Stop", "Waiting for Stop (Log Stopped)" {
          }
          frame "Waiting for Exit (Acq Stopped)" {
            # "If we are waiting to exit, and the acquisition has already stopped, then the \"Logging Stopped\" message indicates that it is time to exit."
            n115 = call-poly "Enqueue Message.vi"("Priority Message? (F)"=TRUE, "error in (no error)"=w324, "Message"="Exit", "Message Queue"=w322) -> ("error out"=w323:errorcluster)  [unwired: 6 in, 1 out]
          }
          frame "Waiting for Stop (Acq Stopped)" {
            # "If we are waiting to stop, and the acquisition has already stopped, then the \"Logging Stopped\" message indicates that it is time to stop."
            n116 = call-poly "Enqueue Message.vi"("error in (no error)"=w330, "Message Data"="Ready..." ("Message"), "Message"="Update Status", "Message Queue"=w328) -> ("error out"=w329:errorcluster)  [unwired: 6 in, 1 out]
          }
        }
      }
      frame "Start" {
        # "Start the loops. In this case we could\n just do a straight start since there is \nonly one loop"
        # "Clear chart"
        # "Message Acquisition and Logging loops to start"
        # "Enable: Stop\nDisable: Start, Exit, Settings"
        # "Start - Enable/Disable buttons appropriately for an acquisition that has started, and update status display."
        n117 = Unbundle By Name(w339) -> ("Trigger Ref"=w350:refnum<vi>, "Stop Ref"=w351:refnum<vi>, "Start Ref"=w354:refnum<vi>, "Exit Ref"=w353:refnum<vi>, "Settings Ref"=w352:refnum<vi>, "Data Ref"=w341:refnum<vi>)
        n118 = property class="WFChart (strict)"(reference=w341, "History Data"=waveform(dbl)[][] []) -> ()  [unwired: 1 in, 2 out]
        n119 = Build Array(w354, w353, w352) -> (w357:refnum<vi>[])
        n120 = Build Array(w350, w351) -> (w356:refnum<vi>[])
        n121 = call-poly "Enqueue Message.vi"("error in (no error)"=w342, "Message"="Broadcast settings", "Message Queue"=w344) -> ("error out"=w345:errorcluster, "dup Message Queue"=w343:refnum<queue>)  [unwired: 7 in]
        n122 = call "Set Enable State on Multiple Controls.vi"("Enable?"=TRUE, "Controls"=w356) -> ()  [unwired: 10 in]
        n123 = call "Set Enable State on Multiple Controls.vi"("Enable?"=FALSE, "Controls"=w357) -> ()  [unwired: 10 in]
        n124 = call-poly "Enqueue Message.vi"("error in (no error)"=w345, "Message"="Start Loops", "Message Queue"=w343) -> ("error out"=w346:errorcluster)  [unwired: 7 in, 1 out]
        n125 = Merge Errors(w346) -> (w333:errorcluster)
        n126 = disable-structure shown="Enabled" {
          disable-tunnel: w338 -> [w359 _]
          frame Disabled {
            n127 = Unbundle By Name(w359) -> ()  [unwired: 1 out]
          }
          frame Enabled {
          }
        }
        n128 = Bundle By Name(cluster=w338, "State"=State_Enum."Measuring") -> (w332:T7)
        n129 = Unbundle By Name(w332) -> ("Process Name"=w336:string)
        n130 = Concatenate Strings(w336, " Start" ("text")) -> (w334:string)
        n131 = call "Write to Log File.vi"("error in"=w333, "text"=w334) -> ()  [unwired: 9 in, 1 out]
      }
      frame "Sequence Start" {
        # "Clear chart"
        # "Message Acquisition and Logging loops to start"
        # "Enable: Stop\nDisable: Start, Exit, Settings"
        # "Start - Enable/Disable buttons appropriately for an acquisition that has started, and update status display."
        n132 = Unbundle By Name(w372) -> ("Trigger Ref"=w379:refnum<vi>, "Stop Ref"=w380:refnum<vi>, "Start Ref"=w383:refnum<vi>, "Exit Ref"=w382:refnum<vi>, "Settings Ref"=w381:refnum<vi>, "Data Ref"=w374:refnum<vi>)
        n133 = property class="WFChart (strict)"(reference=w374, "History Data"=waveform(dbl)[][] []) -> ()  [unwired: 1 in, 2 out]
        n134 = Build Array(w383, w382, w381) -> (w386:refnum<vi>[])
        n135 = Build Array(w379, w380) -> (w385:refnum<vi>[])
        n136 = call-poly "Enqueue Message.vi"("error in (no error)"=w375, "Message"="Broadcast settings", "Message Queue"=w376) -> ("error out"=w368:errorcluster, "dup Message Queue"=w367:refnum<queue>)  [unwired: 7 in]
        n137 = call "Set Enable State on Multiple Controls.vi"("Enable?"=TRUE, "Controls"=w385) -> ()  [unwired: 10 in]
        n138 = call "Set Enable State on Multiple Controls.vi"("Enable?"=FALSE, "Controls"=w386) -> ()  [unwired: 10 in]
        n139 = case shown="False" w365 {
          selector: w365 -> [_ w393]
          tunnel: [w392 w393] -> w369
          tunnel: w368 -> [w391 w394]
          tunnel: w367 -> [w389 _]
          tunnel: [w388 w394] -> w366
          frame False {
            w392 = TRUE  # Sequence Started
            # "Start the loops. In this case we could\n just do a straight start since there is \nonly one loop"
            # "Start the sequence loops"
            n140 = call-poly "Enqueue Message.vi"("error in (no error)"=w391, "Message"="Start Loops", "Message Queue"=w389) -> ("error out"=w388:errorcluster)  [unwired: 7 in, 1 out]
          }
          frame True {
            # "Sequence already started"
          }
        }
        n141 = Merge Errors(w366) -> (w364:errorcluster)
        n142 = Bundle By Name(cluster=w371, "State"=State_Enum."Measuring") -> (w361:T7)
        n143 = Unbundle By Name(w361) -> ("Process Name"=w363:string)
        n144 = Concatenate Strings(w363, " Sequence Start" ("text")) -> (w360:string)
        n145 = call "Write to Log File.vi"("error in"=w364, "text"=w360) -> ()  [unwired: 9 in, 1 out]
      }
      frame "Start Loops" {
        # "Start gets us going"
        # "Message Acquisition and Logging loops to start"
        # "Start - Enable/Disable buttons appropriately for an acquisition that has started, and update status display."
        n146 = Unbundle By Name(w400) -> ("D-O Module Config.Process Name"=w401:string, "D-O Module Config.Settings.Run?"=w395:bool)
        n147 = property class="VI"("Front Panel.Title"=w401) -> ()  [unwired: 2 in, 2 out]
        n148 = call-poly "Enqueue Message.vi"("error in (no error)"=w402, "Message Data"=w401, "Message"="Start", "Message Queue"=w403) -> ("error out"=w398:errorcluster, "dup Message Queue"=w396:refnum<queue>)  [unwired: 6 in]
        n149 = case shown="False" w395 {
          tunnel: w398 -> [w409 w411]
          tunnel: [w408 w411] -> w397
          tunnel: w396 -> [w407 _]
          frame False {
            # "If we are supposed to be paused we pause immediatly"
            n150 = call-poly "Enqueue Message.vi"("error in (no error)"=w409, "Message"="Pause", "Message Queue"=w407) -> ("error out"=w408:errorcluster)  [unwired: 7 in, 1 out]
          }
          frame True {
          }
        }
        n151 = Merge Errors(w397) -> (w406:errorcluster)
      }
      frame "Start Log" {
        # "Message Acquisition and Logging loops to start"
        # "Start - Enable/Disable buttons appropriately for an acquisition that has started, and update status display."
        n152 = Unbundle By Name(w412) -> ("D-O Module Config.Process Name"=w417:string)
        n153 = Build Array(w421) -> (w419:refnum<queue>[])
        n154 = for {
          tunnel: w418 -> [w427]
          tunnel: [w426] -> w420 mode=indexing
          tunnel: w419 -> [w425] mode=indexing
          tunnel: w417 -> [w424]
          n155 = call-poly "Enqueue Message.vi"("error in (no error)"=w427, "Message Data"=w424, "Message"="Start Log", "Message Queue"=w425) -> ("error out"=w426:errorcluster)  [unwired: 6 in, 1 out]
        }
        n156 = property class="VI"("Front Panel.Title"=w417) -> ()  [unwired: 2 in, 2 out]
        n157 = Merge Errors(w420) -> (w416:errorcluster)
        n158 = Unbundle By Name(w412) -> ("Process Name"=w415:string)
        n159 = Concatenate Strings(w415, " Log Started" ("text")) -> (w413:string)
        n160 = call "Write to Log File.vi"("error in"=w416, "text"=w413) -> ()  [unwired: 9 in, 1 out]
      }
      frame "Stop" {
        # "Stop Pauses"
        # "Enable: Start, Exit, Settings\nDisable: Stop"
        # "Stop - Enable/Disable buttons appropriately for an acquisition that has stopped, and update status display."
        n161 = Unbundle By Name(w456) -> ("Trigger Ref"=w447:refnum<vi>, "Stop Ref"=w448:refnum<vi>, "Start Ref"=w451:refnum<vi>, "Exit Ref"=w450:refnum<vi>, "Settings Ref"=w449:refnum<vi>)
        n162 = call-poly "Enqueue Message.vi"("error in (no error)"=w438, "Message"="Broadcast settings", "Message Queue"=w436) -> ("error out"=w437:errorcluster, "dup Message Queue"=w435:refnum<queue>)  [unwired: 7 in]
        n163 = Build Array(w451, w450, w449) -> (w454:refnum<vi>[])
        n164 = Build Array(w447, w448) -> (w453:refnum<vi>[])
        n165 = call-poly "Enqueue Message.vi"("error in (no error)"=w437, "Message Data"="Ready..." ("Ready..."), "Message"="Update Status", "Message Queue"=w435) -> ("error out"=w443:errorcluster)  [unwired: 6 in, 1 out]
        n166 = call "Set Enable State on Multiple Controls.vi"("Enable?"=FALSE, "Controls"=w453) -> ()  [unwired: 10 in]
        n167 = call "Set Enable State on Multiple Controls.vi"("Enable?"=TRUE, "Controls"=w454) -> ()  [unwired: 10 in]
        n168 = call-poly "Enqueue Message.vi"("error in (no error)"=w443, "Message"="Pause", "Message Queue"=w444) -> ("error out"=w441:errorcluster)  [unwired: 7 in, 1 out]
        n169 = case shown="\"Waiting for Exit\"" w445 {
          selector: w445 -> [_ w460]
          tunnel: [UI_State."Waiting for Stop" ("UI State") w460] -> w446
          frame Default {
          }
          frame "Waiting for Exit" {
          }
        }
        n170 = Merge Errors(w441) -> (w433:errorcluster)
        n171 = Bundle By Name(cluster=w440, "State"=State_Enum."Paused") -> (w429:T7)
        n172 = Unbundle By Name(w429) -> ("Process Name"=w432:string)
        n173 = Concatenate Strings(w432, " Stopped" ("text")) -> (w430:string)
        n174 = call "Write to Log File.vi"("error in"=w433, "text"=w430) -> ()  [unwired: 9 in, 1 out]
      }
      frame "Update Status" {
        # "Update Display - Convert the message data to a string to display in the Status indicator."
        n175 = Variant To Data(error in=w471, type="", Variant=w470) -> (data=w464:string, error out=w468:errorcluster)
        "Status" <- w464
        n176 = Unbundle By Name(w467) -> ("Trigger Ref"=w463:refnum<vi>, "Stop Ref"=w466:refnum<vi>)
        n177 = property class="Bool"(reference=w466) -> ("DisabledEnum"=w465:T13)  [unwired: 1 in, 2 out]
        n178 = case shown="\"Enabled\"" w465 {
          tunnel: w464 -> [w475 _]
          tunnel: w463 -> [w476 _]
          frame "Enabled" {
            # "Disable the Force Trigger only while we are logging."
            n179 = Build Array(w476) -> (w477:refnum<vi>[])
            n180 = Not Equal?(x="Logging" ("Logging"), y=w475) -> (x != y?=w473:bool)
            n181 = call "Set Enable State on Multiple Controls.vi"("Enable?"=w473, "Controls"=w477) -> ()  [unwired: 10 in]
          }
          frame "Disabled", Default {
          }
        }
        n182 = Merge Errors(w468) -> (w472:errorcluster)
      }
      frame Default {
        # "'Default' case only runs if there is a message that isn't defined in any of the other cases.  Output a programming error."
        n183 = xnode "Error Ring"("parameter 0"=w480) -> ("error out"=w483:errorcluster)
        n184 = Unbundle By Name(w478) -> ("Process Name"=w482:string)
        n185 = Concatenate Strings(w482, " Invalid Message " ("text"), w480) -> (w479:string)
        n186 = call "Write to Log File.vi"("error in"=w483, "text"=w479) -> ()  [unwired: 9 in, 1 out]
      }
    }
    n187 = Unbundle By Name(w36) -> ()  [unwired: 1 out]
    n188 = call "Error Handler - Message Handling Loop.vi"("error in (no error)"=w50, "Message Queue"=w48) -> ("dup error in"=w49:errorcluster)  [unwired: 8 in, 1 out]
  }
  "Sequence Started" <- w8
  n189 = while {
    tunnel: w27 -> [w502]
    tunnel: [w504] -> w34
    shift-right: [w503] -> w29
    shift-left: w32 -> [w508]
    tunnel: [w501] -> w19
    tunnel: w18 -> [w501]
    tunnel: w13 -> [w500]
    shift-right: [w497] -> _
    shift-left: _ -> [w496]
    stop <- w507 stop-if-true
    # "Event Handling Loop"
    n190 = call "Dequeue Message.vi"("timeout in ms (-1)"=50, "Message Queue"=w500) -> ("error out"=w493:errorcluster, "Message Data"=w498:variant, "Message"=w499:string, "dup Message Queue"=w494:refnum<queue>)  [unwired: 6 in]
    n191 = Flush Queue(queue=w494, error in (no error)=w493) -> ()  [unwired: 3 out]
    n192 = case shown="\"Update\"" w499 {
      tunnel: w498 -> [_ w514]
      tunnel: [w509 w510] -> w497
      tunnel: w496 -> [w509 _]
      frame "False", Default {
      }
      frame "Update" {
        # "Update the display"
        n193 = Variant To Data(type=T14 {"D-O State "=0, "Cycle Period"=0.0} ("FM Display"), Variant=w514) -> (data=w513:T14)  [unwired: 1 in, 1 out]
        n194 = Unbundle By Name(w513) -> ("D-O State"=w512:u16, "Cycle Period"=w510:dbl)
        n195 = case shown="1" w512 {
          frame 0 {
            n196 = local write "Ring"(u16 1 ("Ring")) -> ()
          }
          frame 1 {
            "Ring" <- u16 0 ("Ring")
          }
          frame 2, Default {
            n197 = local write "Ring"(u16 2 ("Ring")) -> ()
          }
        }
      }
    }
    n198 = event "Button Handler" shown="[1] Panel Close?" {
      selector: w508 -> [_ _ _ _ _ _]
      dyn-events: [_ _ _ _ _ _] -> w503
      timeout: w497 -> [_ _ _ _ _ _]
      tunnel: [_ _ _ TRUE ("Discard?") _ _] -> w507
      tunnel: w502 -> [w518 w521 w526 w530 w535 _]
      tunnel: [_ w519 w529 _ w537 _] -> w505
      tunnel: [w518 w520 w525 w530 w536 _] -> w506
      event Timeout {
        n199 = event-data() -> ()  [unwired: 1 in, 1 out]
      }
      event Panel Close? {
        w522 = TRUE  # Priority Message
        n200 = event-data() -> ()  [unwired: 1 in, 1 out]
        n201 = call-poly "Enqueue Message.vi"("Priority Message? (F)"=w522, "Message"="Confirm Quit", "Message Queue"=w521) -> ("error out"=w519:errorcluster, "dup Message Queue"=w520:refnum<queue>)  [unwired: 7 in]
        n202 = event-data("Discard?"=TRUE) -> ()  [unwired: 1 in, 1 out]
      }
      event "Exit": Value Change {
        w527 = TRUE  # Priority Message
        # "The UI Message Loop handles sending the Exit message to other loops."
        n203 = event-data() -> ()  [unwired: 1 in, 1 out]
        n204 = call-poly "Enqueue Message.vi"("Priority Message? (F)"=w527, "Message"="Exit", "Message Queue"=w526) -> ("error out"=w529:errorcluster, "dup Message Queue"=w525:refnum<queue>)  [unwired: 7 in]
      }
      event User Event {
        # "The Message Handling Loop processed an \"Exit\" message, which fired this event to stop the Event Handling Loop."
        n205 = event-data() -> ()  [unwired: 1 in, 1 out]
        n206 = local write "Status"("Exit" ("Exit String")) -> ()
      }
      event "Settings Button": Mouse Down {
        n207 = event-data() -> ("PlatMods"=w534:T15)  [unwired: 1 in]
        n208 = Unbundle By Name(w534) -> ("Ctrl"=w533:bool)
        n209 = case shown="True" w533 {
          tunnel: [w541 w542] -> w537
          tunnel: [w540 w543] -> w536
          tunnel: w535 -> [w539 w543]
          frame False {
            n210 = call-poly "Enqueue Message.vi"("Message"="Launch Settings Dialog", "Message Queue"=w539) -> ("error out"=w541:errorcluster, "dup Message Queue"=w540:refnum<queue>)  [unwired: 8 in]
          }
          frame True {
            n211 = property class="VI"("BDWin.Open"=TRUE ("Block Diagram Window:Open")) -> (error out=w542:errorcluster)  [unwired: 2 in, 1 out]
          }
        }
      }
      event Key Down {
        n212 = event-data() -> ("ScanCode"=→"ScanCode":i16)  [unwired: 1 in]
      }
    }
    n213 = call "Error Handler - Event Handling Loop.vi"("error in (no error)"=w505, "Message Queue"=w506) -> ("dup error in"=w504:errorcluster)  [unwired: 8 in, 1 out]
  }
  n214 = call "Main Loop.vi"("error in (no error)"=w2, "Chart Notifier"=w20, "Message Queues"=w11) -> ("error out"=w21:errorcluster)  [unwired: 8 in]
  n215 = Unregister For Events(event registration refnum=w29, error in=w34) -> (error out=w30:errorcluster)
  n216 = Close Reference(reference=w19) -> ()  [unwired: 1 in, 1 out]
  n217 = Merge Errors(w30, w35, w2, w21) -> (w33:errorcluster)
  n218 = call "Destroy User Event - Stop.vi"("error in (no error)"=w33, "User Event - Stop"=w31) -> ()  [unwired: 9 in, 1 out]
